vi "Problem1.12.vi"() -> ()   [LabVIEW 2019]
panel:
  out "Uniform Deviate 1":dbl
  out "Uniform Deviate 2":dbl
  out "g":dbl
  out "s":dbl
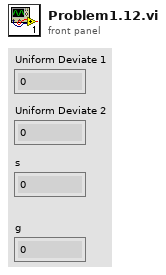
[diagram p1: front panel]
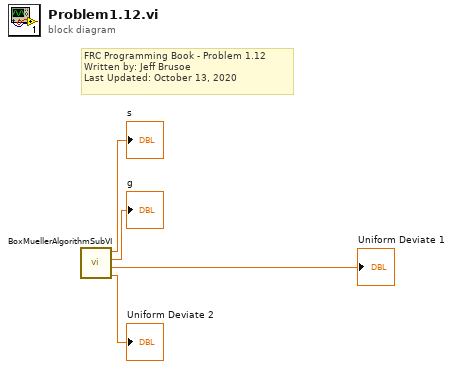
[diagram p0: block diagram]
diagram:
  # "FRC Programming Book - Problem 1.12\nWritten by: Jeff Brusoe\nLast Updated: October 13, 2020"
  n1 = call "BoxMuellerAlgorithmSubVI.vi"() -> ("Uniform Deviate 2"=→"Uniform Deviate 2":dbl, "Uniform Deviate 1"=→"Uniform Deviate 1":dbl, "g"=→"g":dbl, "s"=→"s":dbl)  [unwired: 8 in]
